vi "Linear Fit CI (single)(unused).vi"(8 "error in (no error)":errorcluster, 10 "Type":enum16{"y vs x", "x vs y"}(ring), 11 "XY-data":cluster{"X-array":dbl[], "Y-array":dbl[]}) -> (0 "error out":errorcluster, 2 "Best Fit":cluster{"X-array":dbl[], "Y-array":dbl[]} {"Y-array" format="%.2p"; "X-array" format="%.2p"}, 3 "XY-data out":cluster{"X-array":dbl[], "Y-array":dbl[]})   [LabVIEW 2019, in "xy_utilities.lvlib"]
doc: "Performs numerical differentiation of <b>XY-data</b> using the finite difference method.\n\n<b>Interval</b> is the range over which the finite difference is calculated.\n<b>Interval Units</b> defines the units of the <b>Interval</b> to be the number of points or the same units as the x (or y) data.\n<b>Type</b> specifies taking a derivative with respect to x or y.\n\nWire data to the data input to determine the polymorphic instance to use or manually select the instance."
uses:
  xy_utilities.lvlib
  <vilib>/Analysis/NI_AALPro.lvlib
  Swap X and Y (single).vi
  <vilib>/Analysis/6fits.llb/Confidence Interval (Linear).vi
panel:
  in  "Best Fit":cluster{"X-array":dbl[], "Y-array":dbl[]} {"Y-array" format="%.2p"; "X-array" format="%.2p"}
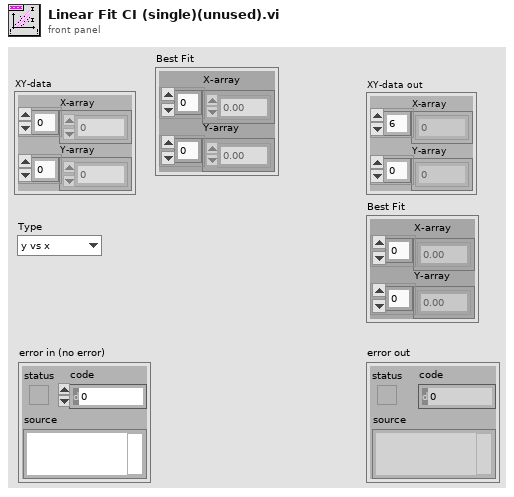
[diagram p1: front panel]
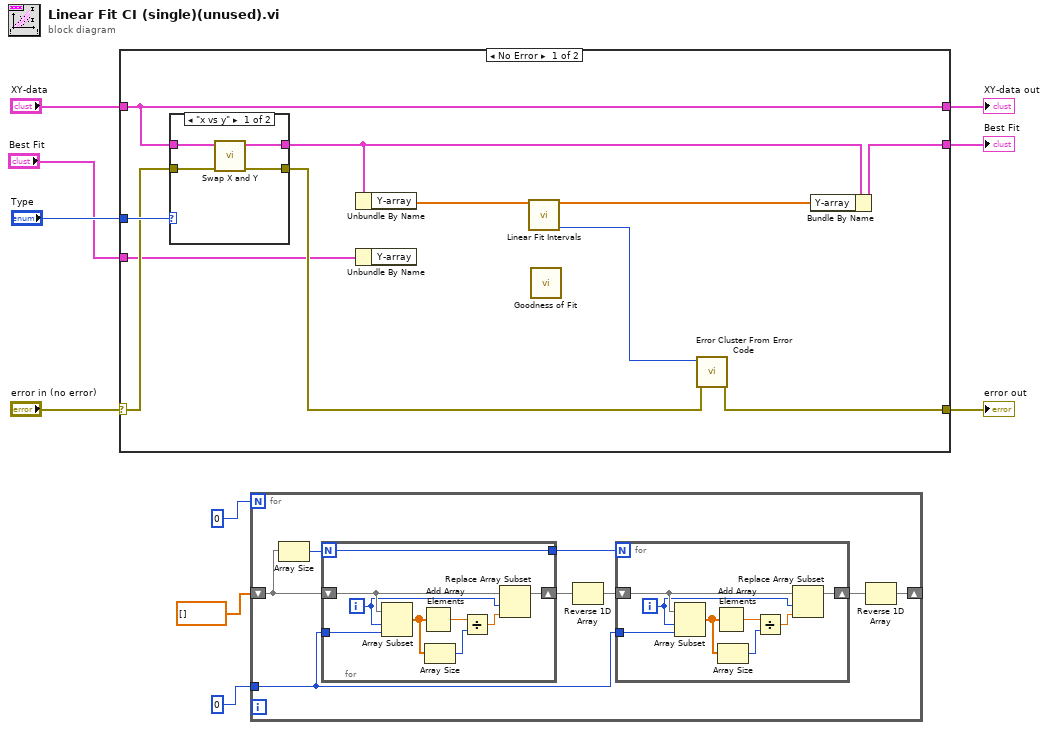
[diagram p0: block diagram]
diagram:
  n1 = case shown="No Error" "error in (no error)" {
    selector: "error in (no error)" -> [w20 w29]
    tunnel: [w16 w29] -> w9
    tunnel: "XY-data" -> [w17 w28]
    tunnel: [w19 _] -> w7
    tunnel: "Type" -> [w21 _]
    tunnel: [w17 w28] -> w5
    tunnel: "Best Fit" -> [w12 _]
    frame No Error {
      n2 = case shown="\"x vs y\"" w21 {
        tunnel: w17 -> [w25 w27]
        tunnel: [w24 w27] -> w18
        tunnel: [w23 w26] -> w15
        tunnel: w20 -> [w22 w26]
        frame "x vs y" {
          n3 = call-poly "Swap X and Y.vi"("error in (no error)"=w22, "XY-data"=w25) -> ("error out"=w23:errorcluster, "XY-data out"=w24:cluster{"X-array":dbl[], "Y-array":dbl[]})  [unwired: 8 in]
        }
        frame "y vs x" {
        }
      }
      n4 = Unbundle By Name(w18) -> ("Y-array"=w14:dbl[])
      n5 = Unbundle By Name(w12) -> ()  [unwired: 1 out]
      n6 = call-poly <vilib>:"Linear Fit Intervals.vi"("Y"=w14) -> ("Upper Bound"=w11:dbl[], "error"=w13:i32)  [unwired: 10 in, 3 out]
      n7 = call <vilib>:"Goodness of Fit.vi"() -> ()  [unwired: 8 in, 4 out]
      n8 = call <vilib>:"Error Cluster From Error Code.vi"("error in (no error)"=w15, "error code (0)"=w13) -> ("error out"=w16:errorcluster)  [unwired: 7 in]
      n9 = Bundle By Name(cluster=w18, "Y-array"=w11) -> (w19:cluster{"X-array":dbl[], "Y-array":dbl[]})
    }
    frame Error {
    }
  }
  "error out" <- w9
  "Best Fit" <- w7
  "XY-data out" <- w5
  n10 = for {
    N: 0 ("iterations") -> [_]
    tunnel: 0 ("Window") -> [w33]
    shift-right: [w32] -> _
    shift-left: dbl[] [] ("Data In") -> [w37]
    n11 = Array Size(array=w37) -> (size(s)=w31:i32)
    n12 = for {
      N: w31 -> [w46]
      shift-right: [w50] -> w36
      shift-left: w37 -> [w53]
      tunnel: w33 -> [w49]
      tunnel: [w46] -> w30
      i -> [w52]
      n13 = Array Subset(array=w53, index=w52, length=w49) -> (w48:dbl[])
      n14 = Add Array Elements(numeric array=w48) -> (sum=w54:dbl)
      n15 = Array Size(array=w48) -> (size(s)=w47:i32)
      n16 = Divide(x=w54, y=w47) -> (x/y=w51:dbl)
      n17 = Replace Array Subset(array=w53, new element=w51, index=w52) -> (w50:dbl[])
    }
    n18 = Reverse 1D Array(array=w36) -> (reversed array=w35:dbl[])
    n19 = for {
      N: w30 -> [_]
      shift-right: [w41] -> w34
      shift-left: w35 -> [w44]
      tunnel: w33 -> [w40]
      i -> [w43]
      n20 = Array Subset(array=w44, index=w43, length=w40) -> (w39:dbl[])
      n21 = Add Array Elements(numeric array=w39) -> (sum=w45:dbl)
      n22 = Array Size(array=w39) -> (size(s)=w38:i32)
      n23 = Divide(x=w45, y=w38) -> (x/y=w42:dbl)
      n24 = Replace Array Subset(array=w44, new element=w42, index=w43) -> (w41:dbl[])
    }
    n25 = Reverse 1D Array(array=w34) -> (reversed array=w32:dbl[])
  }
